vi "monitor2.vi"() -> ()   [LabVIEW 2012]
uses:
  <vilib>/addons/database/Auxilliary.llb/DB Tools Cursor Type.ctl
  <vilib>/addons/database/Connection.llb/DB Tools Open Connec (Path).vi
  <vilib>/addons/database/Connection.llb/Conn Execute.vi
  <vilib>/addons/database/Recordset.llb/Rec Fetch Recordset Data (R).vi
  <vilib>/addons/database/Recordset.llb/Rec Destroy - Connection.vi
  <vilib>/addons/database/_DB Variant To Data/Database Variant To Data.xnode
  <vilib>/addons/database/NI_Database_API.lvlib
panel:
  in  "OK Button":bool
  in  "M100 Monitor Board":string[][](table)
  in  "Table Control":string[][](table)
  in  "input cluster 2":T1
  out "error out 2":errorcluster
  in  "stop":bool
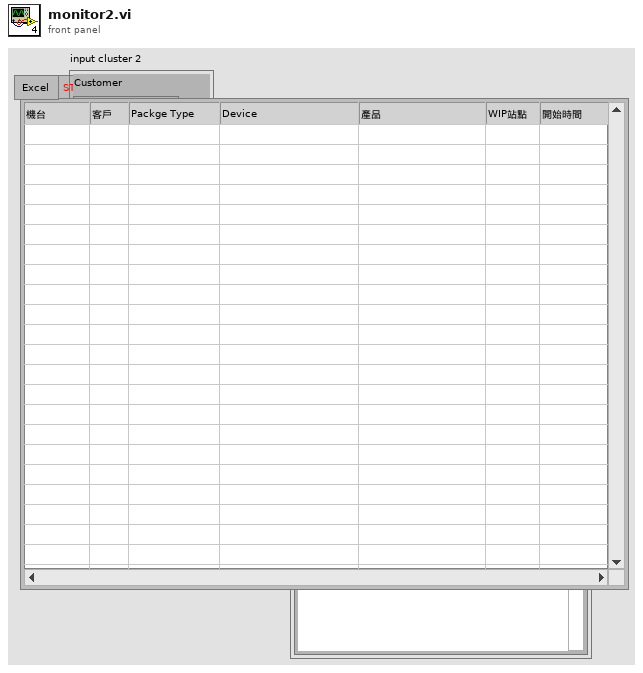
[diagram p1: front panel]
types:
  T1 = cluster{"Customer":string, "Package":string, "machine":string}
  T2 = typedef "NI_Database_API.lvlib/DB Tools Cursor Type.ctl" = enum16{"forward-only", "keyset", "dynamic", "static"}
  T3 = typedef "NI_Database_API.lvlib/Conn ObjectReference.ctl" = refnum<k1>
  T4 = typedef "LVDateTimeRec.ctl" = cluster{"fractional second":dbl, "second":i32, "minute":i32, "hour":i32, "day of month":i32, "month":i32, "year":i32, "day of week":i32, "day of year":i32, "DST":i32}
  T5 = typedef "LVRowAndColumnTypeDef.ctl" = cluster{"Row":i32, "Column":i32}
  T6 = typedef "NI_Database_API.lvlib/Rec ObjectReference.ctl" = refnum<k1>
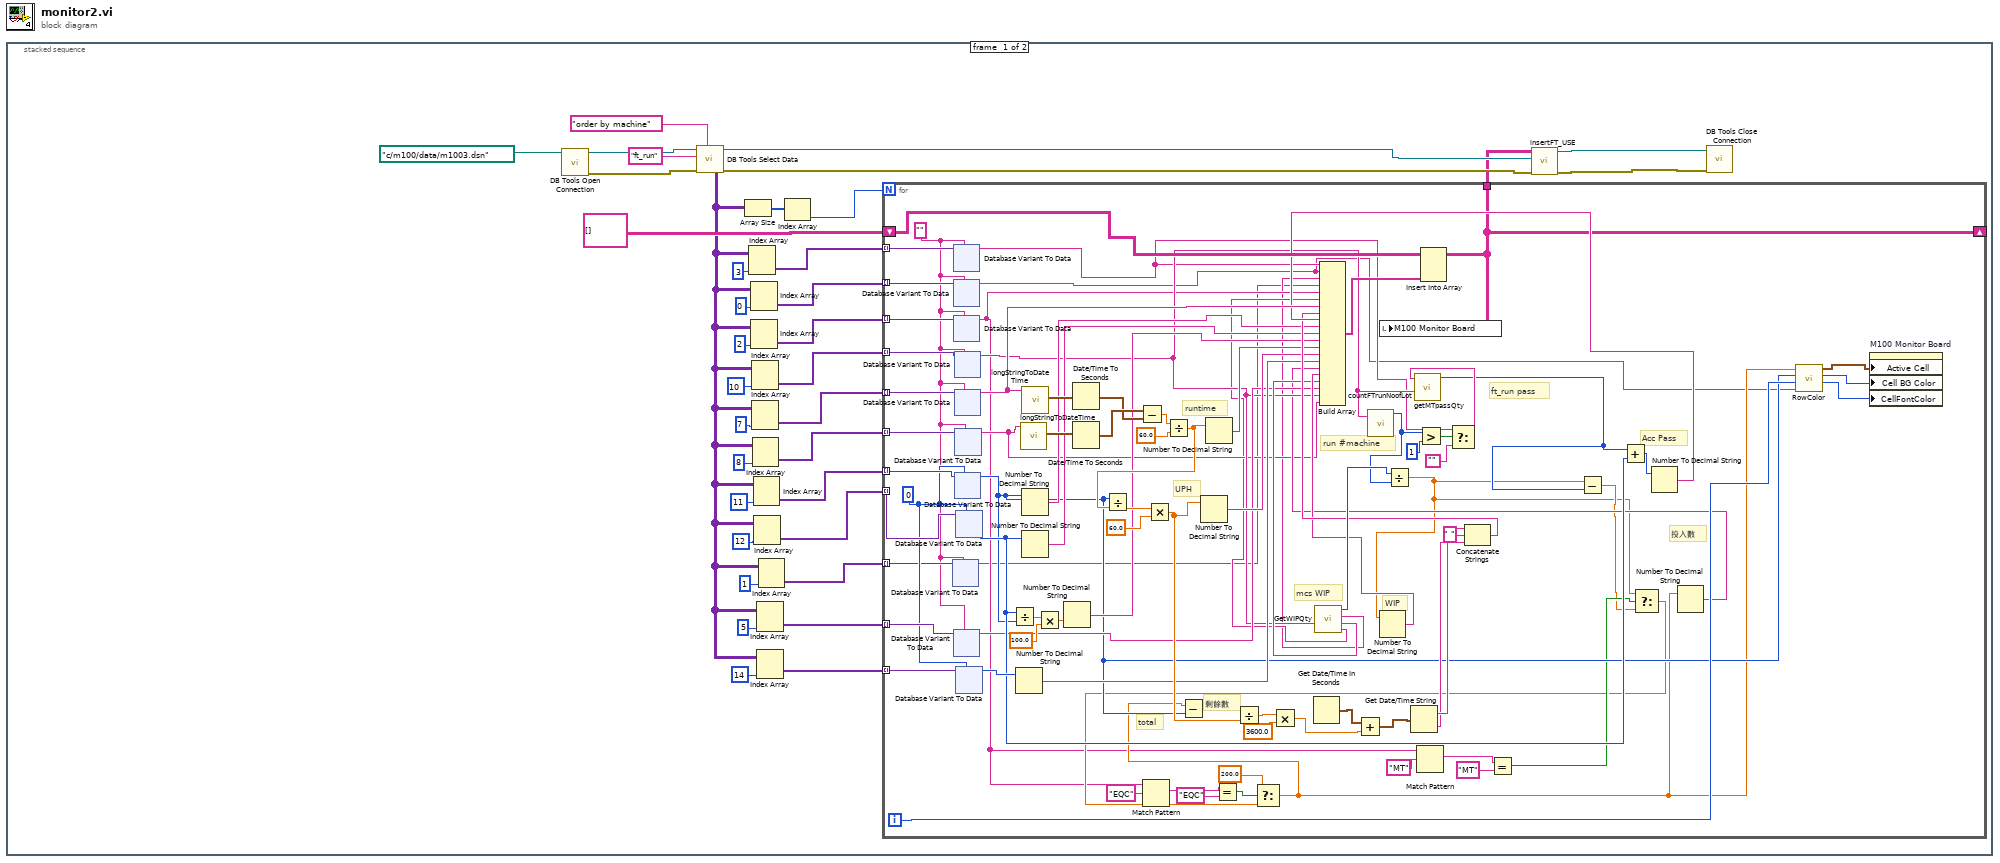
[diagram p0: block diagram]
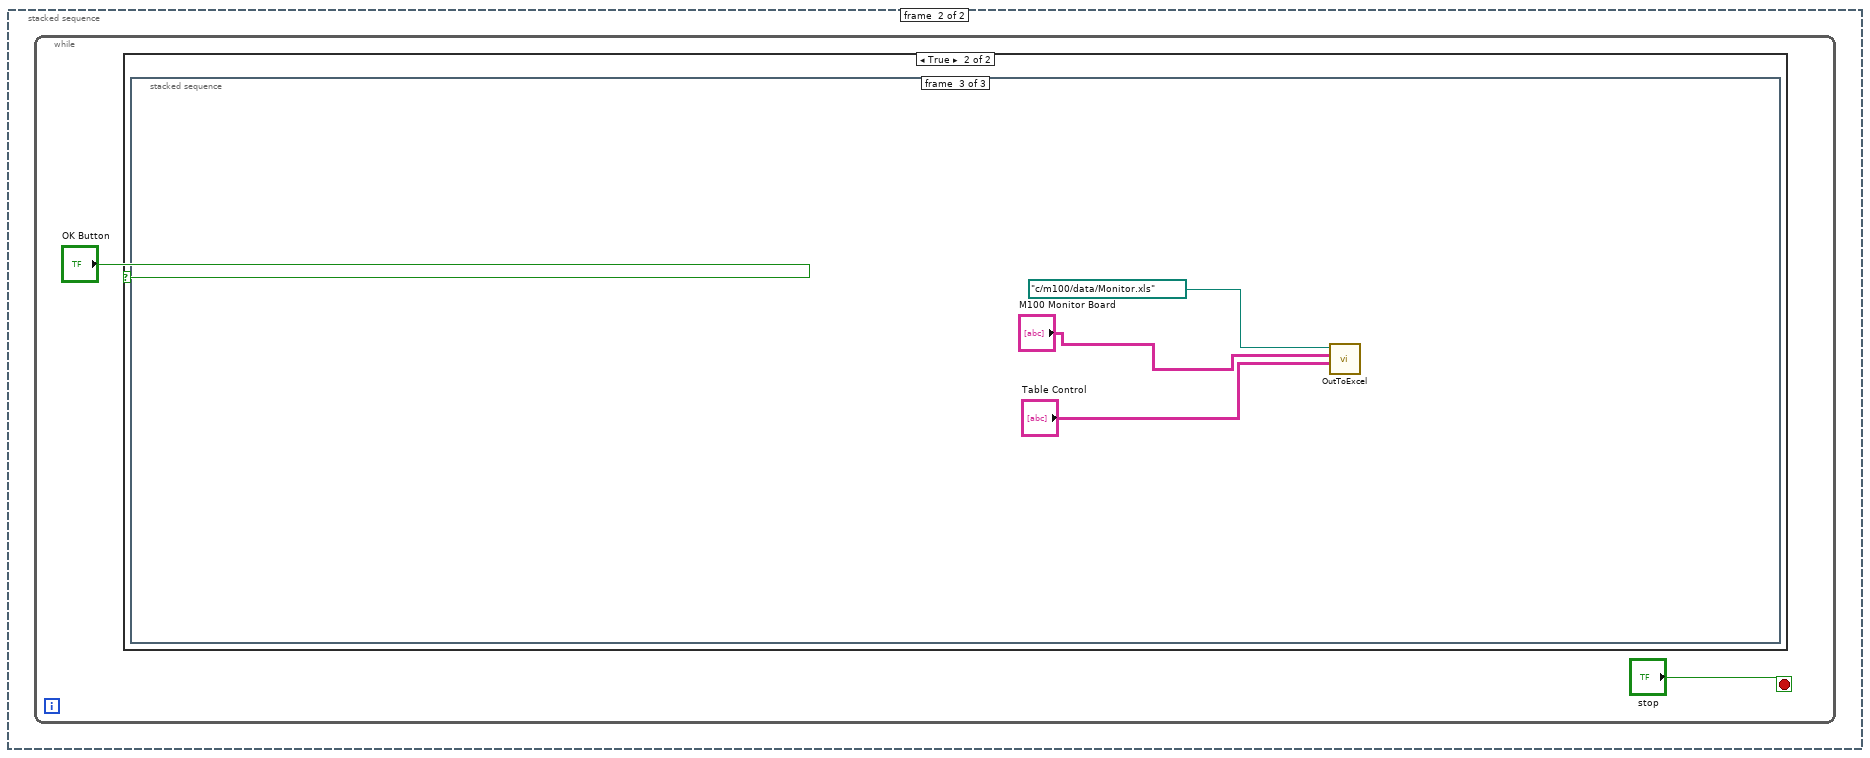
[diagram p2: hidden frame]
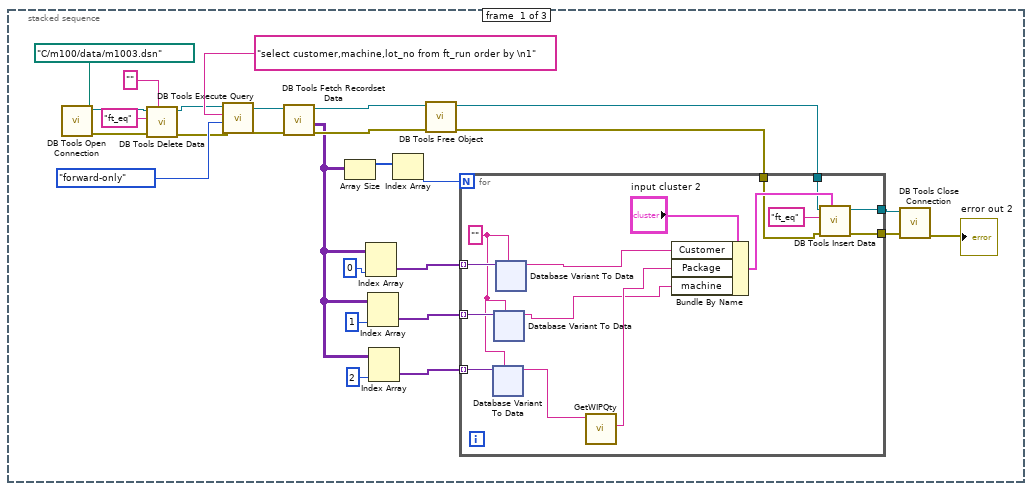
[diagram p4: hidden frame]
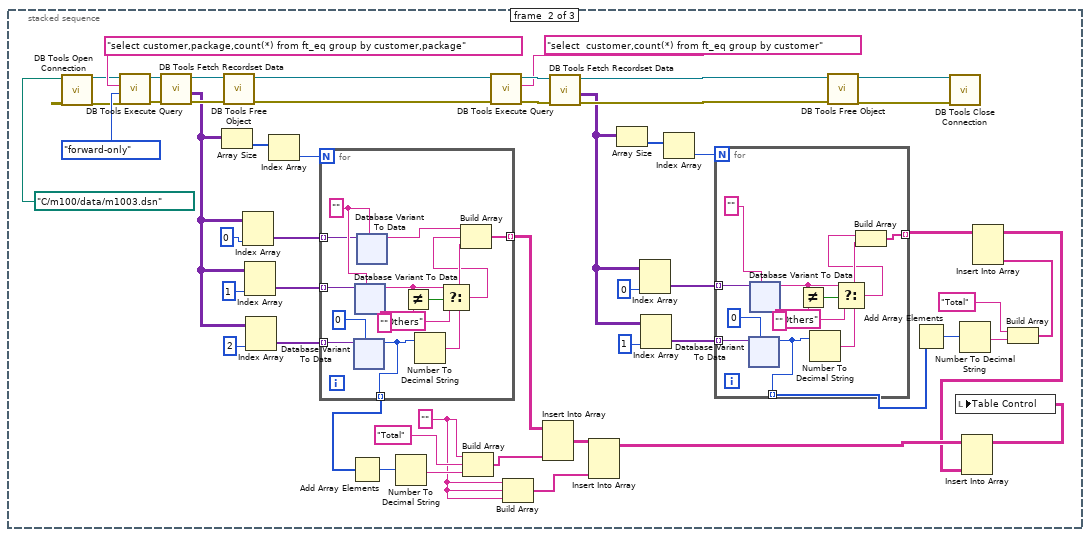
[diagram p5: hidden frame]
diagram:
  n1 = stacked-sequence {
    frame #0 {
      n2 = call-poly <vilib>:"DB Tools Open Connection.vi"("connection information"=path "c:/m100/data/m1003.dsn") -> ("error out"=w35:errorcluster, "connection reference"=w36:T3)  [unwired: 7 in]
      n3 = call <vilib>:"DB Tools Select Data.vi"("condition"="order by machine", "error in (no error)"=w35, "table"="ft_run", "connection reference"=w36) -> ("error out"=w2:errorcluster, "data"=w8:variant[][], "connection reference out"=w3:T3)  [unwired: 2 in]
      n4 = Array Size(array=w8) -> (size(s)=w32:i32[])
      n5 = Index Array(array=w8, index (col)=3) -> (element=w21:variant[])  [unwired: 1 in]
      n6 = Index Array(array=w8, index (col)=0) -> (element=w28:variant[])  [unwired: 1 in]
      n7 = Index Array(array=w8, index (col)=2) -> (element=w20:variant[])  [unwired: 1 in]
      n8 = Index Array(array=w8, index (col)=10) -> (element=w19:variant[])  [unwired: 1 in]
      n9 = Index Array(array=w8, index (col)=7) -> (element=w18:variant[])  [unwired: 1 in]
      n10 = Index Array(array=w8, index (col)=8) -> (element=w14:variant[])  [unwired: 1 in]
      n11 = Index Array(array=w8, index (col)=11) -> (element=w17:variant[])  [unwired: 1 in]
      n12 = Index Array(array=w8, index (col)=12) -> (element=w16:variant[])  [unwired: 1 in]
      n13 = Index Array(array=w8, index (col)=5) -> (element=w12:variant[])  [unwired: 1 in]
      n14 = Index Array(array=w8, index (col)=14 ("disabled index (col)")) -> (element=w10:variant[])  [unwired: 1 in]
      n15 = Index Array(array=w8, index (col)=1 ("disabled index (col)")) -> (element=w6:variant[])  [unwired: 1 in]
      n16 = Index Array(array=w32) -> (element=w31:i32)  [unwired: 1 in]
      n17 = for {
        N: w31 -> [_]
        tunnel: w28 -> [w119] mode=indexing
        tunnel: w16 -> [w123] mode=indexing
        shift-right: [w37] -> _
        shift-left: string[][] [] -> [w122]
        tunnel: w21 -> [w120] mode=indexing
        tunnel: w20 -> [w118] mode=indexing
        tunnel: w19 -> [w117] mode=indexing
        tunnel: w18 -> [w116] mode=indexing
        tunnel: w17 -> [w115] mode=indexing
        tunnel: w14 -> [w111] mode=indexing
        tunnel: w12 -> [w101] mode=indexing
        tunnel: w10 -> [w100] mode=indexing
        tunnel: w6 -> [w45] mode=indexing
        tunnel: [w37] -> w1
        i -> [w85]
        w99 = 0
        w44 = ""
        # "剩餘數"
        # "ft_run pass"
        # "WIP"
        # "mcs WIP"
        # "run #machine"
        # "Acc Pass"
        # "total"
        # "UPH"
        # "runtime"
        # "投入數"
        n18 = xnode "Database Variant To Data"("database variant"=w45, "type"=w44) -> ("data"=w38:string)  [unwired: 1 in, 1 out]
        n19 = xnode "Database Variant To Data"("database variant"=w120, "type"=w44) -> ("data"=w41:string)  [unwired: 1 in, 1 out]
        n20 = xnode "Database Variant To Data"("database variant"=w119, "type"=w44) -> ("data"=w40:string)  [unwired: 1 in, 1 out]
        n21 = xnode "Database Variant To Data"("database variant"=w118, "type"=w44) -> ("data"=w43:string)  [unwired: 1 in, 1 out]
        n22 = xnode "Database Variant To Data"("database variant"=w101, "type"=w44) -> ("data"=w65:string)  [unwired: 1 in, 1 out]
        n23 = xnode "Database Variant To Data"("database variant"=w117, "type"=w44) -> ("data"=w64:string)  [unwired: 1 in, 1 out]
        n24 = xnode "Database Variant To Data"("database variant"=w116, "type"=w44) -> ("data"=w76:string)  [unwired: 1 in, 1 out]
        n25 = xnode "Database Variant To Data"("database variant"=w115, "type"=w99) -> ("data"=w55:i32)  [unwired: 1 in, 1 out]
        n26 = xnode "Database Variant To Data"("database variant"=w111, "type"=w44) -> ("data"=w61:string)  [unwired: 1 in, 1 out]
        n27 = xnode "Database Variant To Data"("database variant"=w123, "type"=w99) -> ("data"=w83:i32)  [unwired: 1 in, 1 out]
        n28 = xnode "Database Variant To Data"("database variant"=w100, "type"=w99) -> ("data"=w98:i32)  [unwired: 1 in, 1 out]
        n29 = Divide(x=w83, y=w55) -> (x/y=w112:dbl)
        n30 = Number To Decimal String(number=w98) -> (decimal integer string=w68:string)  [unwired: 1 in]
        n31 = call "longStringToDateTime.vi"("input string"=w61) -> ("output cluster"=w110:T4)  [unwired: 10 in]
        n32 = call "longStringToDateTime.vi"("input string"=w76) -> ("output cluster"=w109:T4)  [unwired: 10 in]
        n33 = Number To Decimal String(number=w55) -> (decimal integer string=w73:string)  [unwired: 1 in]
        n34 = Number To Decimal String(number=w83) -> (decimal integer string=w72:string)  [unwired: 1 in]
        n35 = Multiply(x=w112, y=100.0) -> (x*y=w113:dbl)
        n36 = Number To Decimal String(number=w113) -> (decimal integer string=w71:string)  [unwired: 1 in]
        n37 = Date/Time To Seconds(2:w109) -> (0:w107:timestamp)  [unwired: 1 in]
        n38 = Date/Time To Seconds(2:w110) -> (0:w108:timestamp)  [unwired: 1 in]
        n39 = Subtract(x=w108, y=w107) -> (x-y=w106:dbl)
        n40 = Match Pattern(string=w43, regular expression="EQC") -> (match substring=w59:string)  [unwired: 1 in, 3 out]
        n41 = Divide(x=w106, y=60.0) -> (x/y=w104:dbl)
        n42 = Divide(x=w55, y=w104) -> (x/y=w103:dbl)
        n43 = Multiply(x=w103, y=60.0) -> (x*y=w97:dbl)
        n44 = Number To Decimal String(number=w97) -> (decimal integer string=w69:string)  [unwired: 1 in]
        n45 = Number To Decimal String(number=w104) -> (decimal integer string=w70:string)  [unwired: 1 in]
        n46 = Equal?(x=w59, y="EQC") -> (x = y?=w57:bool)
        n47 = Get Date/Time In Seconds() -> (seconds since 1Jan1904=w94:timestamp)
        n48 = call "GetWIPQty.vi"("Lotno"=w64) -> ("step"=w42:string, "lotno"=w66:string, "Package"=w39:string, "data"=w84:i32)  [unwired: 7 in]
        n49 = call "countFTrunNoofLot.vi"("Lotno"=w64) -> ("data"=w81:i32)  [unwired: 10 in]
        n50 = Divide(x=w84, y=w81) -> (x/y=w49:dbl)
        n51 = Number To Decimal String(number=w49) -> (decimal integer string=w67:string)  [unwired: 1 in]
        n52 = Match Pattern(string=w43, regular expression="MT") -> (match substring=w53:string)  [unwired: 1 in, 3 out]
        n53 = Greater?(x=w81, y=1) -> (0:w79:bool)
        n54 = Select(t=w41, s=w79, f="") -> (s? t:f=w77:string)
        n55 = call "getMTpassQty.vi"("Lot"=w64, "machine"=w77) -> ("data"=w62:i32)  [unwired: 9 in]
        n56 = Equal?(x=w53, y="MT") -> (x = y?=w51:bool)
        n57 = Subtract(x=w49, y=w62) -> (x-y=w50:dbl)
        n58 = Add(x=w62, y=w83) -> (x+y=w82:i32)
        n59 = Select(t=w49, s=w51, f=w50) -> (s? t:f=w48:dbl)
        n60 = Select(t=200.0, s=w57, f=w48) -> (s? t:f=w46:dbl)
        n61 = Subtract(x=w46, y=w55) -> (x-y=w47:dbl)
        n62 = Divide(x=w47, y=w97) -> (x/y=w96:dbl)
        n63 = Multiply(x=w96, y=3600.0) -> (x*y=w93:dbl)
        n64 = Add(x=w94, y=w93) -> (x+y=w92:timestamp)
        n65 = Get Date/Time String(seconds (now)=w92) -> (date string=w91:string, time string=w90:string)  [unwired: 2 in]
        n66 = Concatenate Strings(w91, " " ("string"), w90) -> (w74:string)
        n67 = Number To Decimal String(number=w82) -> (decimal integer string=w75:string)  [unwired: 1 in]
        n68 = Number To Decimal String(number=w46) -> (decimal integer string=w63:string)  [unwired: 1 in]
        n69 = Build Array(w41, w40, w39, w38, w43, w42, w76, w74, w75, w73, w72, w71, w70, w69, w68, w63, w67, w66, w65, w64, w61) -> (w121:string[])
        n70 = Insert Into Array(array=w122, new element=w121) -> (w37:string[][])  [unwired: 2 in]
        n71 = local write "M100 Monitor Board"(w37) -> ()
        n72 = call "RowColor.vi"("Customer"=w40, "Row"=w85, "tested"=w55, "Input"=w46) -> ("FontColor"=w86:u32, "bgcolor"=w87:u32, "ActiveCell"=w88:T5)  [unwired: 5 in]
        n73 = property on="M100 Monitor Board" class="Tbl (strict)"("Active Cell"=w88, "Cell BG Color"=w87, "CellFontColor"=w86) -> ()  [unwired: 2 in, 2 out]
      }
      n74 = call "insertFT_USE.vi"("M100 Monitor Board"=w1, "connection reference"=w3, "error out 2"=w2) -> ("connection reference out"=w5:T3, "error out"=w4:errorcluster)  [unwired: 6 in]
      n75 = call <vilib>:"DB Tools Close Connection.vi"("error in (no error)"=w4, "connection reference"=w5) -> ()  [unwired: 5 in, 1 out]
    }
    frame #1 {
      n76 = while {
        stop <- "stop" stop-if-true
        n77 = case shown="True" "OK Button" {
          frame False {
          }
          frame True {
            n78 = stacked-sequence {
              frame #0 {
                n79 = call-poly <vilib>:"DB Tools Open Connection.vi"("connection information"=path "C:/m100/data/m1003.dsn") -> ("error out"=w488:errorcluster, "connection reference"=w489:T3)  [unwired: 7 in]
                n80 = call <vilib>:"DB Tools Delete Data.vi"("condition"="", "error in (no error)"=w488, "table"="ft_eq", "connection reference"=w489) -> ("error out"=w486:errorcluster, "connection reference out"=w485:T3)  [unwired: 6 in]
                n81 = call-poly <vilib>:"DB Tools Execute Query.vi"("error in (no error)"=w486, "cursor type"=DB_Tools_Cursor_Type."forward-only", "SQL query"="select customer,machine,lot_no from ft_run order by \n1", "connection reference"=w485) -> ("error out"=w501:errorcluster, "recordset reference"=w503:T6)  [unwired: 4 in]
                n82 = call-poly <vilib>:"DB Tools Fetch Recordset Data.vi"("error in (no error)"=w501, "recordset reference"=w503) -> ("error out"=w500:errorcluster, "recordset data"=w495:variant[][], "recordset reference out"=w502:T6)  [unwired: 3 in]
                n83 = Array Size(array=w495) -> (size(s)=w494:i32[])
                n84 = Index Array(array=w495, index (col)=0 ("disabled index (col)")) -> (element=w492:variant[])  [unwired: 1 in]
                n85 = Index Array(array=w495, index (col)=1 ("disabled index (col)")) -> (element=w491:variant[])  [unwired: 1 in]
                n86 = Index Array(array=w495, index (col)=2) -> (element=w490:variant[])  [unwired: 1 in]
                n87 = Index Array(array=w494) -> (element=w493:i32)  [unwired: 1 in]
                n88 = call-poly <vilib>:"DB Tools Free Object.vi"("error in (no error)"=w500, "recordset reference"=w502) -> ("error out"=w481:errorcluster, "connection reference"=w482:T3)  [unwired: 8 in]
                n89 = for {
                  N: w493 -> [_]
                  tunnel: w492 -> [w519] mode=indexing
                  tunnel: w491 -> [w518] mode=indexing
                  tunnel: w490 -> [w517] mode=indexing
                  tunnel: w482 -> [w508]
                  tunnel: w481 -> [w507]
                  tunnel: [w506] -> w480
                  tunnel: [w505] -> w479
                  w516 = ""
                  n90 = xnode "Database Variant To Data"("database variant"=w517, "type"=w516) -> ("data"=w515:string)  [unwired: 1 in, 1 out]
                  n91 = xnode "Database Variant To Data"("database variant"=w518, "type"=w516) -> ("data"=w510:string)  [unwired: 1 in, 1 out]
                  n92 = xnode "Database Variant To Data"("database variant"=w519, "type"=w516) -> ("data"=w512:string)  [unwired: 1 in, 1 out]
                  n93 = call "GetWIPQty.vi"("Lotno"=w515) -> ("Package"=w511:string)  [unwired: 7 in, 3 out]
                  n94 = Bundle By Name(cluster="input cluster 2", "Customer"=w512, "Package"=w511, "machine"=w510) -> (w509:T1)
                  n95 = call <vilib>:"DB Tools Insert Data.vi"("data"=w509, "error in (no error)"=w507, "table"="ft_eq", "connection reference"=w508) -> ("error out"=w505:errorcluster, "connection reference out"=w506:T3)  [unwired: 6 in]
                }
                n96 = call <vilib>:"DB Tools Close Connection.vi"("error in (no error)"=w479, "connection reference"=w480) -> ("error out"=→"error out 2":errorcluster)  [unwired: 5 in]
              }
              frame #1 {
                w625 = "" ("element")
                n97 = call-poly <vilib>:"DB Tools Open Connection.vi"("connection information"=path "C:/m100/data/m1003.dsn") -> ("error out"=w654:errorcluster, "connection reference"=w655:T3)  [unwired: 7 in]
                n98 = call-poly <vilib>:"DB Tools Execute Query.vi"("error in (no error)"=w654, "cursor type"=DB_Tools_Cursor_Type."forward-only", "SQL query"="select customer,package,count(*) from ft_eq group by customer,package", "connection reference"=w655) -> ("error out"=w664:errorcluster, "recordset reference"=w666:T6)  [unwired: 4 in]
                n99 = call-poly <vilib>:"DB Tools Fetch Recordset Data.vi"("error in (no error)"=w664, "recordset reference"=w666) -> ("error out"=w663:errorcluster, "recordset data"=w658:variant[][], "recordset reference out"=w665:T6)  [unwired: 3 in]
                n100 = Array Size(array=w658) -> (size(s)=w657:i32[])
                n101 = call-poly <vilib>:"DB Tools Free Object.vi"("error in (no error)"=w663, "recordset reference"=w665) -> ("error out"=w622:errorcluster, "connection reference"=w623:T3)  [unwired: 8 in]
                n102 = Index Array(array=w658, index (col)=0 ("disabled index (col)")) -> (element=w652:variant[])  [unwired: 1 in]
                n103 = Index Array(array=w658, index (col)=1 ("disabled index (col)")) -> (element=w651:variant[])  [unwired: 1 in]
                n104 = Index Array(array=w658, index (col)=2) -> (element=w650:variant[])  [unwired: 1 in]
                n105 = Index Array(array=w657) -> (element=w653:i32)  [unwired: 1 in]
                n106 = for {
                  N: w653 -> [_]
                  tunnel: w652 -> [w756] mode=indexing
                  tunnel: w651 -> [w755] mode=indexing
                  tunnel: w650 -> [w754] mode=indexing
                  tunnel: [w750] -> w645 mode=indexing
                  tunnel: [w744] -> w648 mode=indexing
                  w757 = ""
                  n107 = xnode "Database Variant To Data"("database variant"=w754, "type"=0) -> ("data"=w744:i32)  [unwired: 1 in, 1 out]
                  n108 = xnode "Database Variant To Data"("database variant"=w755, "type"=w757) -> ("data"=w747:string)  [unwired: 1 in, 1 out]
                  n109 = xnode "Database Variant To Data"("database variant"=w756, "type"=w757) -> ("data"=w752:string)  [unwired: 1 in, 1 out]
                  n110 = Not Equal?(x=w747, y="") -> (x != y?=w748:bool)
                  n111 = Number To Decimal String(number=w744) -> (decimal integer string=w751:string)  [unwired: 1 in]
                  n112 = Select(t=w747, s=w748, f="Others") -> (s? t:f=w745:string)
                  n113 = Build Array(w752, w745, w751) -> (w750:string[])
                }
                n114 = Add Array Elements(numeric array=w648) -> (sum=w649:i32)
                n115 = Number To Decimal String(number=w649) -> (decimal integer string=w647:string)  [unwired: 1 in]
                n116 = Build Array(w625, "Total" ("element"), w647) -> (w644:string[])
                n117 = call-poly <vilib>:"DB Tools Execute Query.vi"("error in (no error)"=w622, "SQL query"="select  customer,count(*) from ft_eq group by customer", "connection reference"=w623) -> ("error out"=w641:errorcluster, "recordset reference"=w643:T6)  [unwired: 5 in]
                n118 = Build Array(w625, w625, w625) -> (w624:string[])
                n119 = Insert Into Array(array=w645, new element=w644) -> (w626:string[][])  [unwired: 2 in]
                n120 = call-poly <vilib>:"DB Tools Fetch Recordset Data.vi"("error in (no error)"=w641, "recordset reference"=w643) -> ("error out"=w640:errorcluster, "recordset data"=w637:variant[][], "recordset reference out"=w642:T6)  [unwired: 3 in]
                n121 = Insert Into Array(array=w626, new element=w624) -> (w618:string[][])  [unwired: 2 in]
                n122 = Array Size(array=w637) -> (size(s)=w636:i32[])
                n123 = Index Array(array=w637, index (col)=0 ("disabled index (col)")) -> (element=w634:variant[])  [unwired: 1 in]
                n124 = Index Array(array=w637, index (col)=1) -> (element=w633:variant[])  [unwired: 1 in]
                n125 = Index Array(array=w636) -> (element=w635:i32)  [unwired: 1 in]
                n126 = for {
                  N: w635 -> [_]
                  tunnel: w634 -> [w678] mode=indexing
                  tunnel: w633 -> [w677] mode=indexing
                  tunnel: [w674] -> w628 mode=indexing
                  tunnel: [w668] -> w631 mode=indexing
                  n127 = xnode "Database Variant To Data"("database variant"=w677, "type"=0) -> ("data"=w668:i32)  [unwired: 1 in, 1 out]
                  n128 = xnode "Database Variant To Data"("database variant"=w678, "type"="") -> ("data"=w671:string)  [unwired: 1 in, 1 out]
                  n129 = Not Equal?(x=w671, y="") -> (x != y?=w672:bool)
                  n130 = Number To Decimal String(number=w668) -> (decimal integer string=w675:string)  [unwired: 1 in]
                  n131 = Select(t=w671, s=w672, f="Others") -> (s? t:f=w669:string)
                  n132 = Build Array(w669, w675) -> (w674:string[])
                }
                n133 = call-poly <vilib>:"DB Tools Free Object.vi"("error in (no error)"=w640, "recordset reference"=w642) -> ("error out"=w620:errorcluster, "connection reference"=w621:T3)  [unwired: 8 in]
                n134 = Add Array Elements(numeric array=w631) -> (sum=w632:i32)
                n135 = call <vilib>:"DB Tools Close Connection.vi"("error in (no error)"=w620, "connection reference"=w621) -> ()  [unwired: 5 in, 1 out]
                n136 = Number To Decimal String(number=w632) -> (decimal integer string=w630:string)  [unwired: 1 in]
                n137 = Build Array("Total" ("element"), w630) -> (w627:string[])
                n138 = Insert Into Array(array=w628, new element=w627) -> (w617:string[][])  [unwired: 2 in]
                n139 = Insert Into Array(array=w618, new element=w617) -> (w616:string[][])  [unwired: 2 in]
                n140 = local write "Table Control"(w616) -> ()
              }
              frame #2 {
                n141 = call "OutToExcel.vi"("Table Control"="Table Control", "Running"="M100 Monitor Board", "Report Template"=path "c:/m100/data/Monitor.xls") -> ()  [unwired: 9 in]
              }
            }
          }
        }
      }
    }
  }
